vi "AC_CmdStr_2F1.vi"(1 "AC命令输入":T1 {"驻车空调失效状态" items=["失效", "未失效", "预留"]; "驻车空调状态" items=["关闭", "开启", "预留", "无效"]; "PM2.5传感器工作状态" items=["初始态", "数据收集中", "完成", "关闭"]; "室内空气质量等级" items=["Level1", "Level2", "Level3", "Level4", "Level5", "Level6", "预留", "无效"]; "室外空气PM2.5浓度" min=0 max=999 step=1 scale=0.0..999.0; "室内空气PM2.5浓度" min=0 max=999 step=1 scale=0.0..999.0; "AC大气温度传感器读数" min=-40.0 max=60.0 step=0.5 scale=-40.0..60.0}) -> (0 "CmdStr":string)   [LabVIEW 2013]
uses:
  AC_2F1.ctl
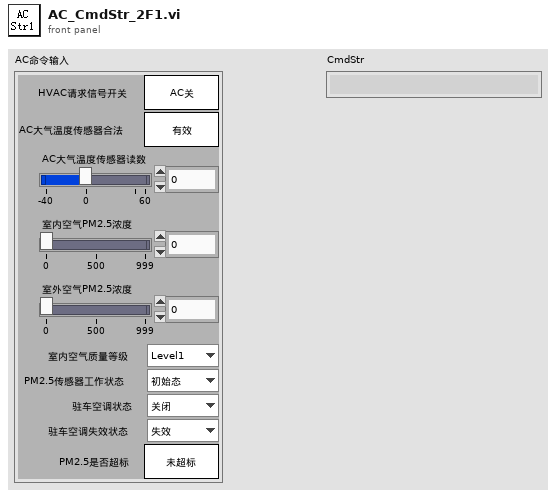
[diagram p1: front panel]
types:
  T1 = typedef "AC_2F1.ctl" = cluster{"HVAC请求信号开关":bool, "AC大气温度传感器合法":bool, "AC大气温度传感器读数":dbl, "室内空气PM2.5浓度":i32, "室外空气PM2.5浓度":i32, "室内空气质量等级":u16, "PM2.5传感器工作状态":u16, "驻车空调状态":u16, "驻车空调失效状态":u16, "PM2.5是否超标":bool}
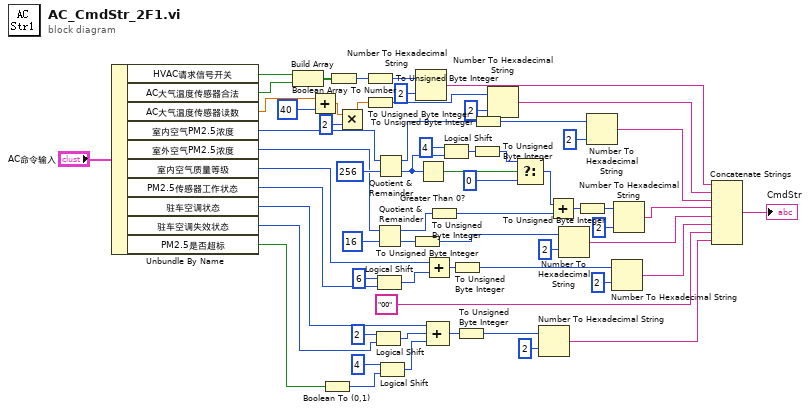
[diagram p0: block diagram]
diagram:
  n1 = Unbundle By Name("AC命令输入") -> ("HVAC请求信号开关"=w62:bool, "AC大气温度传感器合法"=w61:bool, "AC大气温度传感器读数"=w58:dbl, "室内空气PM2.5浓度"=w43:i32, "室外空气PM2.5浓度"=w42:i32, "室内空气质量等级"=w38:u16, "PM2.5传感器工作状态"=w40:u16, "驻车空调状态"=w33:u16, "驻车空调失效状态"=w35:u16, "PM2.5是否超标"=w31:bool)
  n2 = Build Array(w62, w61) -> (w60:bool[])
  n3 = Add(x=w58, y=u8 40) -> (x+y=w4:dbl)
  n4 = Boolean To (0,1)(Boolean=w31) -> (0, 1=w30:i16)
  n5 = Boolean Array To Number(Boolean array=w60) -> (number=w59:u32)
  n6 = Multiply(x=w4, y=2) -> (x*y=w2:dbl)
  n7 = To Unsigned Byte Integer(number=w59) -> (unsigned 8bit integer=w26:u8)
  n8 = To Unsigned Byte Integer(number=w2) -> (unsigned 8bit integer=w23:u8)
  n9 = Logical Shift(y=u8 2, x=w35) -> (x << y=w34:u16)
  n10 = Logical Shift(y=u8 6, x=w40) -> (x << y=w39:u16)
  n11 = Quotient & Remainder(x=w42, y=16) -> (x-y*floor(x/y)=w45:i32, floor(x/y)=w46:i32)
  n12 = Quotient & Remainder(x=w43, y=256) -> (x-y*floor(x/y)=w48:i32, floor(x/y)=w51:i32)
  n13 = Logical Shift(y=u8 4, x=w30) -> (x << y=w28:i16)
  n14 = To Unsigned Byte Integer(number=w46) -> (unsigned 8bit integer=w13:u8)
  n15 = Number To Hexadecimal String(1:2, 2:w26) -> (0:w25:string)
  n16 = Greater Than 0?(x=w51) -> (x > 0?=w55:bool)
  n17 = Add(x=w38, y=w39) -> (x+y=w37:u16)
  n18 = Compound Arithmetic op=ADD(w33, w34, w28) -> (w32:u16)
  n19 = To Unsigned Byte Integer(number=w45) -> (unsigned 8bit integer=w44:u8)
  n20 = Logical Shift(y=u8 4, x=w51) -> (x << y=w53:i32)
  n21 = To Unsigned Byte Integer(number=w37) -> (unsigned 8bit integer=w8:u8)
  n22 = To Unsigned Byte Integer(number=w32) -> (unsigned 8bit integer=w5:u8)
  n23 = To Unsigned Byte Integer(number=w53) -> (unsigned 8bit integer=w49:u8)
  n24 = To Unsigned Byte Integer(number=w48) -> (unsigned 8bit integer=w20:u8)
  n25 = Number To Hexadecimal String(1:2, 2:w23) -> (0:w24:string)
  n26 = Select(t=w49, s=w55, f=u8 0) -> (s? t:f=w47:u8)
  n27 = Number To Hexadecimal String(1:2, 2:w5) -> (0:w6:string)
  n28 = Add(x=w47, y=w44) -> (x+y=w14:u8)
  n29 = Number To Hexadecimal String(1:2, 2:w13) -> (0:w12:string)
  n30 = To Unsigned Byte Integer(number=w14) -> (unsigned 8bit integer=w17:u8)
  n31 = Number To Hexadecimal String(1:2, 2:w20) -> (0:w19:string)
  n32 = Number To Hexadecimal String(1:2, 2:w8) -> (0:w9:string)
  n33 = Number To Hexadecimal String(1:2, 2:w17) -> (0:w16:string)
  n34 = Concatenate Strings(w25, w24, w19, w16, w12, w9, "00", w6) -> (→"CmdStr":string)
